vi "InitializeTrackingParameters.vi"(0 "Rectangular selection":T1 {"Rotation" format="%.2f"; "Left" scale=0.0..1024.0; "Right" scale=0.0..1024.0}, 1 "Cancel":bool, 2 "Circle fit parameters in":T2) -> (4 "Pupil Marked":bool, 6 "Circle fit parameters out":T2)   [LabVIEW 2013]
doc: "InitializeEyeTrackerData creates a pop up for making a crop on the video of the pupil and outputs a cluster with parameters for circular fitting, and an array for storing results.\n\nInput\nRefnum In - An image from the video acquisition to choose a cropped region from\n\nOutput\nCircle fit parameters (cluster of 5 elements)\n - Frame No (int) - Number of the current frame\n - Circle Time series (array) - A table for storing results from circle fitting, e.g frame no, radius and x and y coordinates for center position\n - Rectangle coordinates (array) - Rectangle coordinates for the cropped region of the picture\n - Annulus ROI (cluster) - An annulus ROI from the imaq package\n - Annulus coordinates (array) - Annulus coordinates of the Annulus ROI"
uses:
  TrackingParameters.ctl
panel:
  # "This VI creates creates rois for searching for the pupil and outputs a cluster with parameters for circular fitting, and an array for storing results.\n\n\nOutput\nCircle fit parameters\nFrame No (int) - Number of the current frame\nCircle Time series (array) -  A table for storing results from circle fitting, e.g frame no, radius and x and y coordinates for center position\nRectangle coordinates (array) - Rectangle coordinates for the cropped region of the picture\nAnnulus ROI (cluster) - An annulus ROI from the imaq package\nAnnulus coordinates (array) - Annulus coordinates of the Annulus ROI"
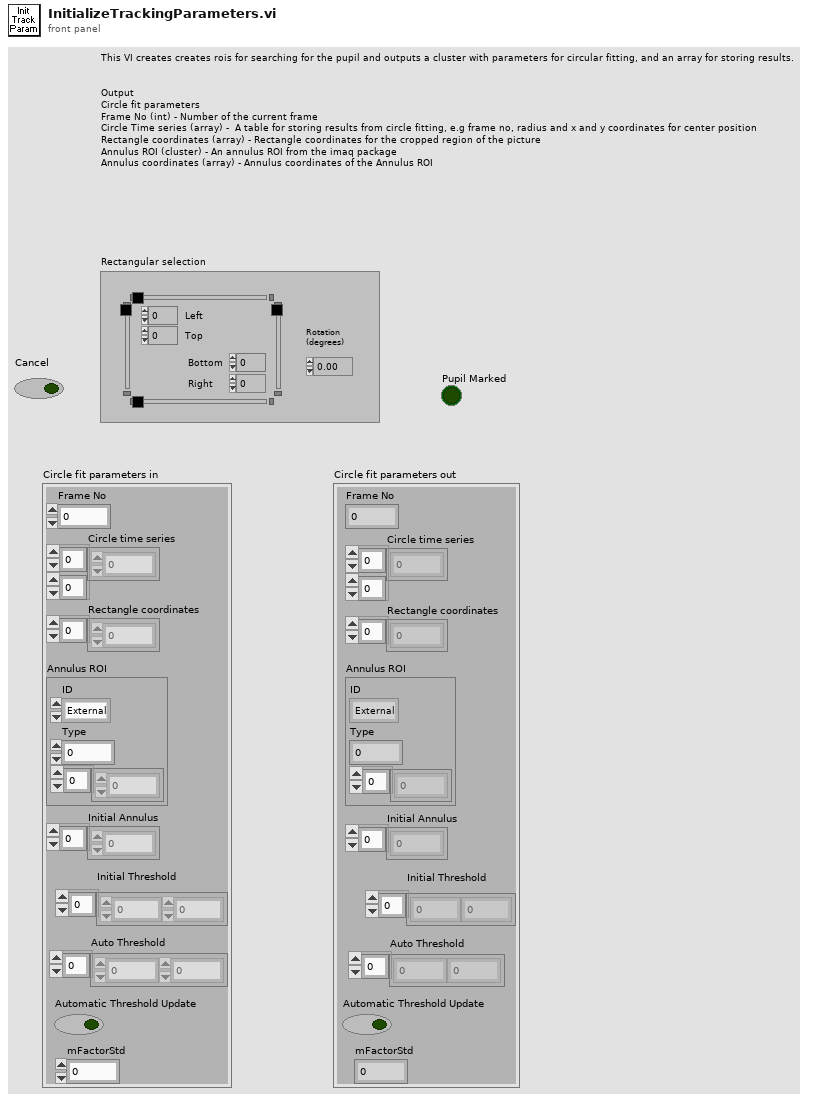
[diagram p1: front panel]
types:
  T1 = typedef "IMAQ Rectangle" = cluster{"Left":i32, "Top":i32, "Right":i32, "Bottom":i32, "Rotation":dbl}
  T2 = typedef "TrackingParameters.ctl" = cluster{"Frame No":i32, "Circle time series":dbl[][], "Rectangle coordinates":i32[], "Annulus ROI":cluster{"ID":enum32{"External", "Internal"}, "Type":u32, i32[]}, "Initial Annulus":i32[], "Auto Threshold":sgl[], "Automatic Threshold Update":bool, "Initial Threshold":sgl[], "mFactorStd":dbl}
  T3 = cluster{"ID":enum32{"External", "Internal"}, "Type":u32, "Coordinates":i32[]}
  T4 = typedef "IMAQ Circle" = cluster{"Center X":i32, "Center Y":i32, "Inner Radius":i32, "Outer Radius":i32, "Start Angle":dbl, "End Angle":dbl}
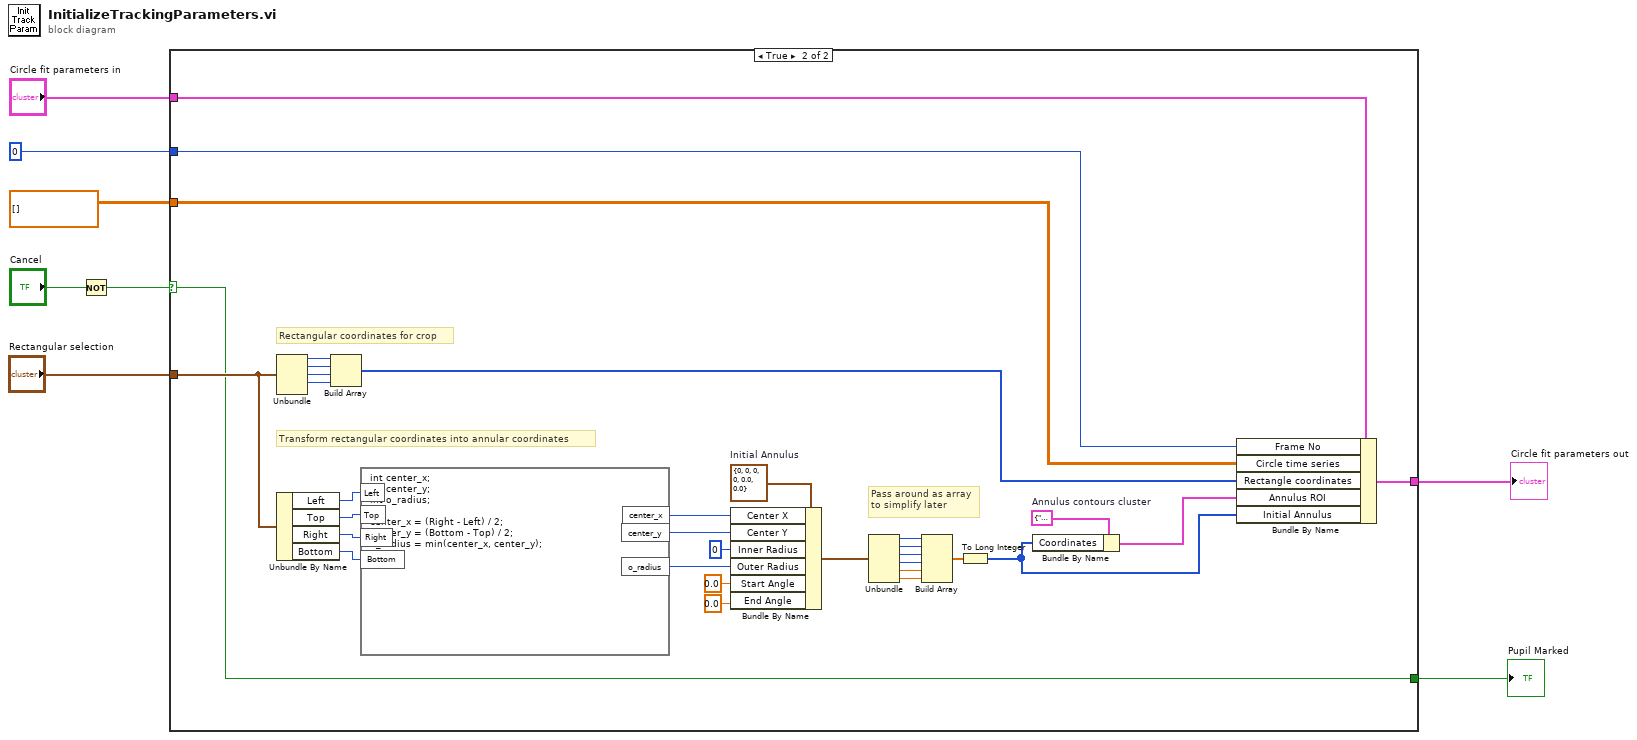
[diagram p0: block diagram]
diagram:
  n1 = Not(x="Cancel") -> (.not. x?=w2:bool)
  n2 = case shown="True" w2 {
    selector: w2 -> [w10 w12]
    tunnel: [w9 w43] -> w1
    tunnel: dbl[][] [] -> [_ w37]
    tunnel: 0 ("Frame No") -> [_ w36]
    tunnel: "Rectangular selection" -> [_ w31]
    tunnel: "Circle fit parameters in" -> [w9 w11]
    tunnel: [w10 w12] -> w5
    frame False {
    }
    frame True {
      w30 = T3 {"ID"=enum."External", "Type"=7, "Coordinates"=[]}  # Annulus contours cluster
      w35 = T4 {"Center X"=0, "Center Y"=0, "Inner Radius"=0, "Outer Radius"=0, "Start Angle"=0.0, "End Angle"=0.0}  # Initial Annulus
      # "Transform rectangular coordinates into annular coordinates"
      # "Pass around as array\nto simplify later"
      # "Rectangular coordinates for crop"
      n3 = Unbundle(w31) -> ("Left"=w40:i32, "Top"=w42:i32, "Right"=w39:i32, "Bottom"=w41:i32)  [unwired: 1 out]
      n4 = Unbundle By Name(w31) -> ("Left"=w21:i32, "Top"=w20:i32, "Right"=w19:i32, "Bottom"=w18:i32)
      n5 = Build Array(w40, w42, w39, w41) -> (w38:i32[])
      n6 = formula code="int center_x;\nint center_y;\nint o_radius;\n\ncenter_x = (Right - Left) / 2;\ncenter_y = (Bottom - Top) / 2;\no_radius = min(center_x, center_y);"("Left"=w21, "Top"=w20, "Right"=w19, "Bottom"=w18) -> ("center_x"=w17:i32, "center_y"=w16:i32, "o_radius"=w15:i32)
      n7 = Bundle By Name(cluster=w35, "Center X"=w17, "Center Y"=w16, "Inner Radius"=0, "Outer Radius"=w15, "Start Angle"=0.0, "End Angle"=0.0) -> (w28:T4)
      n8 = Unbundle(w28) -> ("Center X"=w27:i32, "Center Y"=w26:i32, "Inner Radius"=w24:i32, "Outer Radius"=w25:i32, "Start Angle"=w23:dbl, "End Angle"=w22:dbl)
      n9 = Build Array(w27, w26, w24, w25, w23, w22) -> (w14:dbl[])
      n10 = To Long Integer(number=w14) -> (32bit integer=w13:i32[])
      n11 = Bundle By Name(cluster=w30, "Coordinates"=w13) -> (w29:T3)
      n12 = Bundle By Name(cluster=w11, "Frame No"=w36, "Circle time series"=w37, "Rectangle coordinates"=w38, "Annulus ROI"=w29, "Initial Annulus"=w13) -> (w43:T2)
    }
  }
  "Circle fit parameters out" <- w1
  "Pupil Marked" <- w5
